vi "UDMA_READ_FIFO.vi"(0 "TCP Network Connection in":refnum<k5>, 2 "N":u32=100, 5 "error in (no error)":errorcluster) -> (14 "TCP Network Connection out":refnum<k5>, 16 "Oscilloscope":u32[](graph), 18 "Status Flag":u32, 19 "error out":errorcluster)   [LabVIEW 2020]
panel:
  out "N":u32
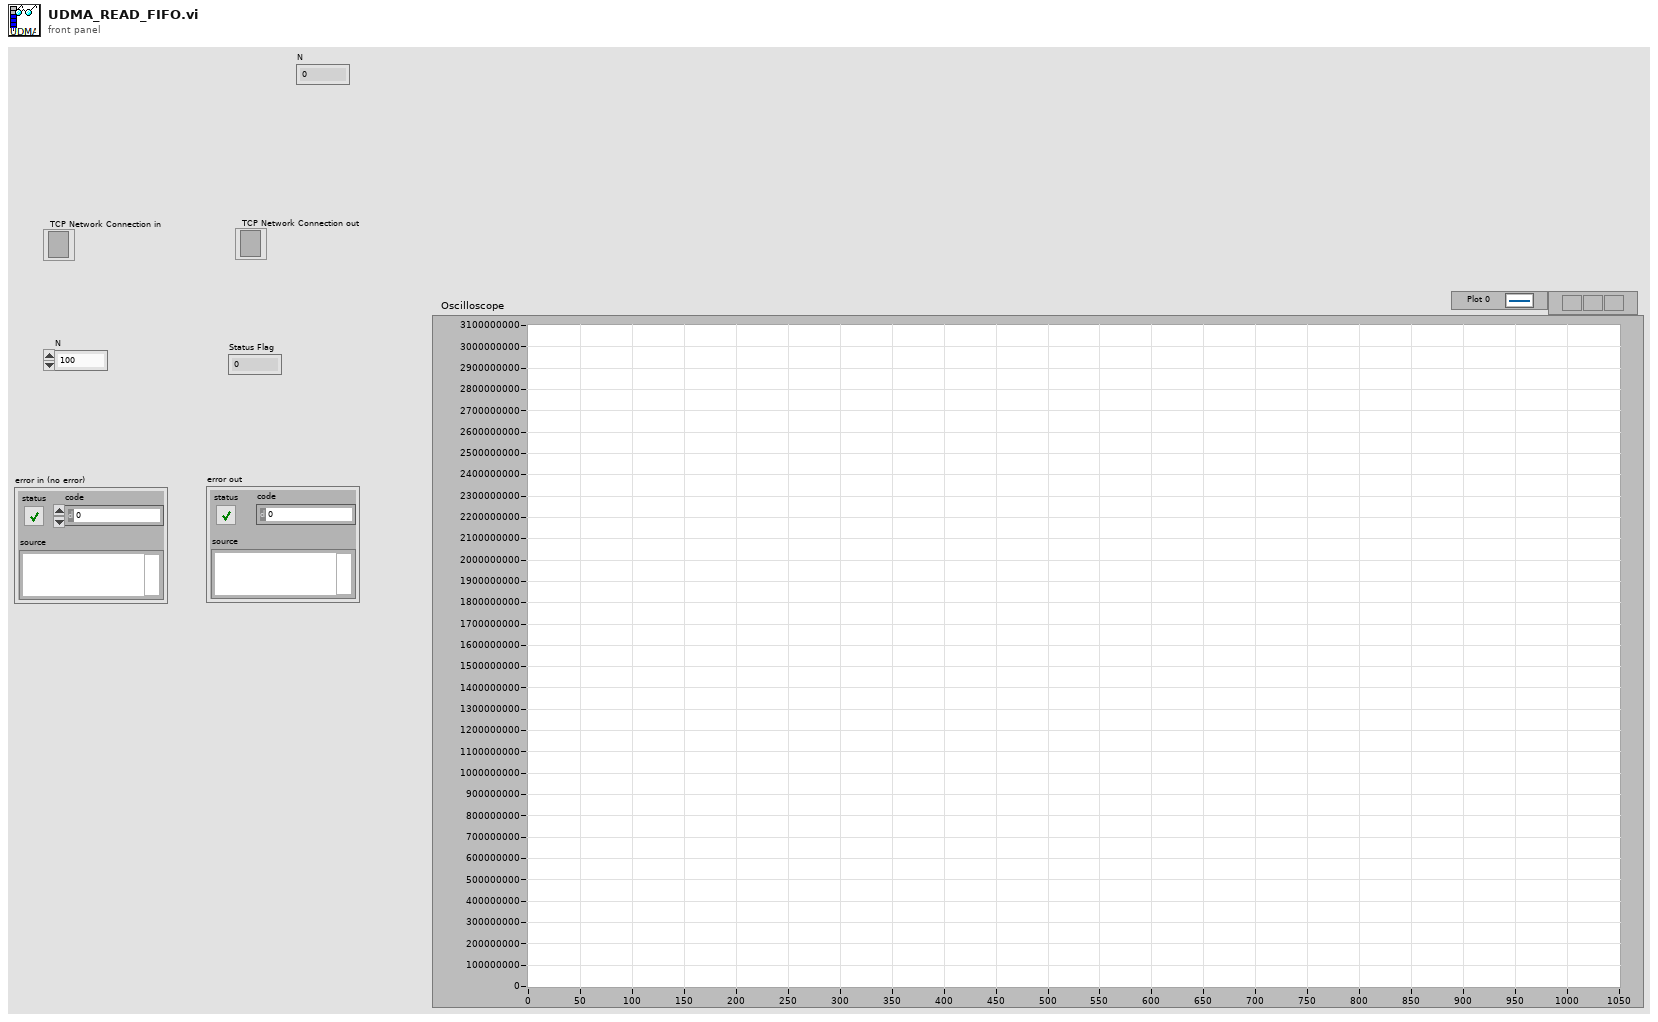
[diagram p1: front panel]
types:
  T1 = enum16{"big-endian, network order", "native, host order", "little-endian"}
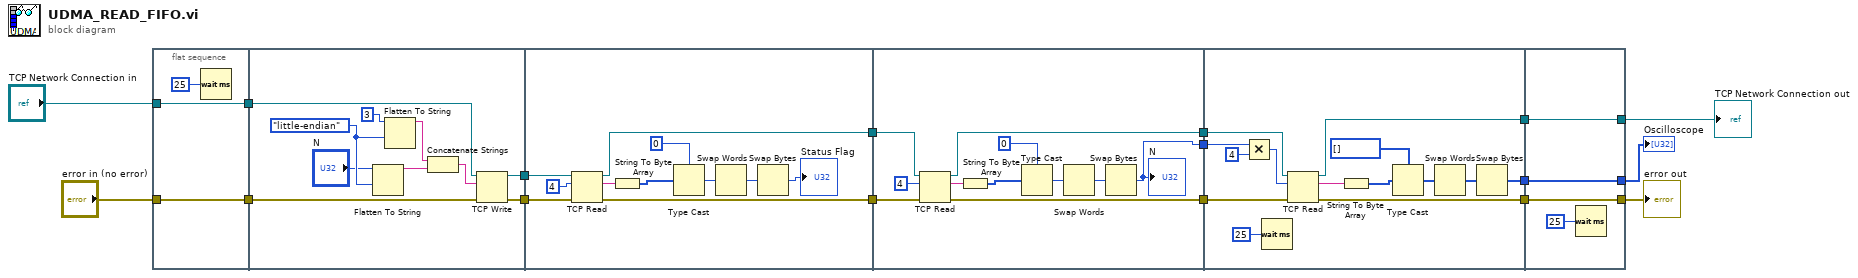
[diagram p0: block diagram]
diagram:
  n1 = flat-sequence {
    tunnel: [w19] -> w13
    tunnel: [w20] -> w12
    tunnel: "error in (no error)" -> [w20]
    tunnel: "TCP Network Connection in" -> [w19]
    tunnel: w13 -> [w30]
    tunnel: w12 -> [w29]
    tunnel: [w28] -> w4
    tunnel: [w27] -> w3
    tunnel: w4 -> [w35]
    tunnel: w3 -> [w34]
    tunnel: [w33] -> w2
    tunnel: [w32] -> w1
    tunnel: w2 -> [w52]
    tunnel: [w51] -> w7
    tunnel: [w42] -> w6
    tunnel: [w50] -> w5
    tunnel: w1 -> [w49]
    tunnel: w7 -> [w65]
    tunnel: w6 -> [w55]
    tunnel: [w64] -> w10
    tunnel: [w63] -> w9
    tunnel: [w53] -> w8
    tunnel: w5 -> [w66]
    tunnel: [w68] -> w11
    tunnel: [w69] -> w15
    tunnel: [w70] -> w14
    tunnel: w10 -> [w70]
    tunnel: w9 -> [w69]
    tunnel: w8 -> [w68]
    frame #0 {
      n2 = Wait (ms)(milliseconds to wait=u32 25) -> ()  [unwired: 1 out]
    }
    frame #1 {
      w25 = T1."little-endian" ("byte order (0:big-endian, network order)")
      n3 = Flatten To String(anything="N", byte order (0:big-endian, network order)=w25) -> (data string=w26:string)  [unwired: 2 in, 2 out]
      n4 = Flatten To String(anything=u32 3 ("element"), byte order (0:big-endian, network order)=w25) -> (data string=w23:string)  [unwired: 2 in, 2 out]
      n5 = Concatenate Strings(w23, w26) -> (w22:string)
      n6 = TCP Write(connection ID=w30, data in=w22, error in (no error)=w29) -> (connection ID out=w28:refnum<k5>, error out=w27:errorcluster)  [unwired: 1 in, 1 out]
    }
    frame #2 {
      n7 = TCP Read(connection ID=w35, bytes to read=4, error in (no error)=w34) -> (connection ID out=w32:refnum<k5>, data out=w41:string, error out=w33:errorcluster)  [unwired: 2 in]
      n8 = String To Byte Array(string=w41) -> (unsigned byte array=w39:u8[])
      n9 = Type Cast(type=u32 0 ("y"), x=w39) -> (*(type *) &x=w38:u32)
      n10 = Swap Words(1:w38) -> (0:w37:u32)
      n11 = Swap Bytes(anything=w37) -> (byte swapped=→"Status Flag":u32)
    }
    frame #3 {
      n12 = TCP Read(connection ID=w49, bytes to read=4, error in (no error)=w52) -> (connection ID out=w50:refnum<k5>, data out=w48:string, error out=w51:errorcluster)  [unwired: 2 in]
      n13 = String To Byte Array(string=w48) -> (unsigned byte array=w46:u8[])
      n14 = Type Cast(type=u32 0 ("y"), x=w46) -> (*(type *) &x=w45:u32)
      n15 = Swap Words(1:w45) -> (0:w44:u32)
      n16 = Swap Bytes(anything=w44) -> (byte swapped=w42:u32)
      "N" <- w42
    }
    frame #4 {
      n17 = Multiply(x=w55, y=u32 4) -> (x*y=w61:u32)
      n18 = Wait (ms)(milliseconds to wait=u32 25) -> ()  [unwired: 1 out]
      n19 = TCP Read(connection ID=w66, bytes to read=w61, error in (no error)=w65) -> (connection ID out=w64:refnum<k5>, data out=w54:string, error out=w63:errorcluster)  [unwired: 2 in]
      n20 = String To Byte Array(string=w54) -> (unsigned byte array=w59:u8[])
      n21 = Type Cast(type=u32[] [], x=w59) -> (*(type *) &x=w57:u32[])
      n22 = Swap Words(1:w57) -> (0:w56:u32[])
      n23 = Swap Bytes(anything=w56) -> (byte swapped=w53:u32[])
    }
    frame #5 {
      n24 = Wait (ms)(milliseconds to wait=u32 25) -> ()  [unwired: 1 out]
    }
  }
  "error out" <- w15
  "TCP Network Connection out" <- w14
  "Oscilloscope" <- w11
